vi "UpdateSettingsCluster(ValueField).vi"(8 "error in (no error)":errorcluster, 9 "SubClusterName":string, 10 "Value":variant, 11 "Picomotor8742 in":refnum<class "Picomotor8742.lvclass">) -> (0 "error out":errorcluster, 3 "Picomotor8742 out":refnum<class "Picomotor8742.lvclass">)   [LabVIEW 2020, in "Picomotor8742.lvclass"]
uses:
  Picomotor8742.lvclass
panel:
  out "Success?":bool
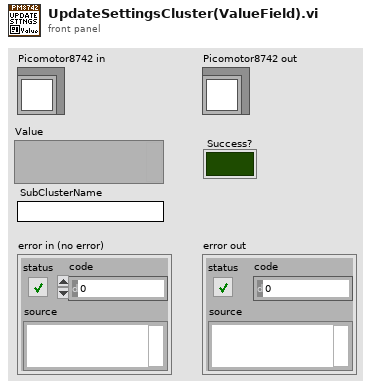
[diagram p1: front panel]
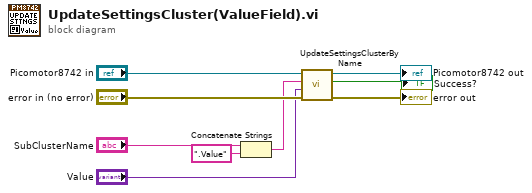
[diagram p0: block diagram]
diagram:
  n1 = Concatenate Strings("SubClusterName", ".Value" ("string")) -> (w5:string)
  n2 = call-dynamic "UpdateSettingsClusterByName.vi"("error in (no error)"="error in (no error)", "ElementValue"="Value", "ElementLabel"=w5, "Picomotor8742 in"="Picomotor8742 in") -> ("error out"=→"error out":errorcluster, "Success?"=→"Success?":bool, "Picomotor8742 out"=→"Picomotor8742 out":refnum<class "Picomotor8742.lvclass">)  [unwired: 5 in]
